vi "Configure Smoothing.vi"(5 "Smoothing State (F: Off)":bool, 7 "Channel (1)":i32=1, 8 "error in (no error)":errorcluster, 10 "Factor (1.5)":dbl=1.5 format="%01_3g", 11 "VISA resource name":refnum<visa-resource-name>) -> (0 "error out":errorcluster, 3 "VISA resource name out":refnum<visa-resource-name>)   [LabVIEW 2023, in "Agilent ENA Series.lvlib"]
doc: "Configures the smoothing for active channel."
uses:
  Agilent ENA Series.lvlib
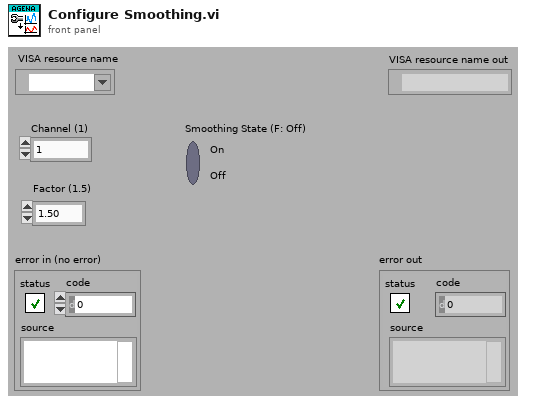
[diagram p1: front panel]
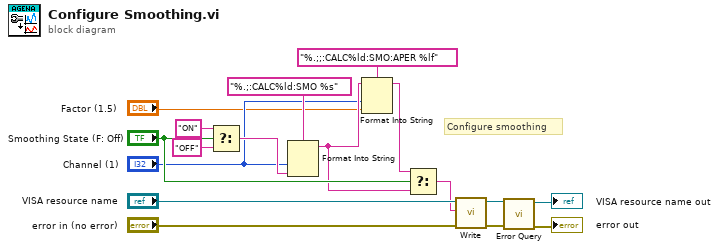
[diagram p0: block diagram]
diagram:
  # "Configure smoothing"
  n1 = Select(t="ON", s="Smoothing State (F: Off)", f="OFF") -> (s? t:f=w12:string)
  n2 = Format Into String(format string="%.;:CALC%ld:SMO %s", "Channel (1)", w12) -> (resulting string=w7:string)  [unwired: 2 in, 1 out]
  n3 = Format Into String(format string="%.;;:CALC%ld:SMO:APER %lf", initial string=w7, "Channel (1)", "Factor (1.5)") -> (resulting string=w9:string)  [unwired: 1 in, 1 out]
  n4 = Select(t=w9, s="Smoothing State (F: Off)", f=w7) -> (s? t:f=w8:string)
  n5 = call "Write.vi"("error in (no error)"="error in (no error)", "String ()"=w8, "VISA resource name"="VISA resource name") -> ("error out"=w3:errorcluster, "VISA resource name out"=w4:refnum<visa-resource-name>)  [unwired: 6 in, 1 out]
  n6 = call "Error Query.vi"("error in (no error)"=w3, "VISA resource name"=w4) -> ("error out"=→"error out":errorcluster, "VISA resource name out"=→"VISA resource name out":refnum<visa-resource-name>)  [unwired: 6 in, 2 out]
